vi "testSourceTree2.vi"() -> ()   [LabVIEW 2018]
panel:
  out "数値: 0から1":dbl
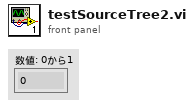
[diagram p1: front panel]
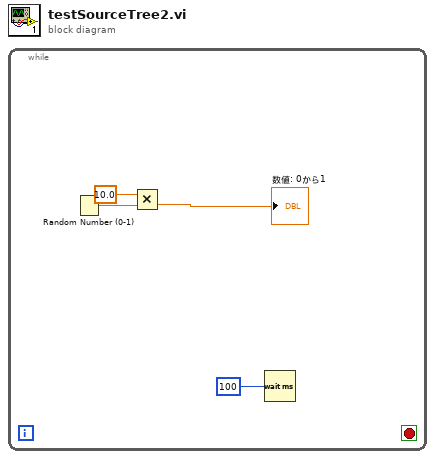
[diagram p0: block diagram]
diagram:
  n1 = while {
    stop <- _ stop-if-true
    n2 = Random Number (0-1)() -> (number: 0 to 1=w4:dbl)
    n3 = Multiply(x=10.0, y=w4) -> (x*y=→"数値: 0から1":dbl)
    n4 = Wait (ms)(milliseconds to wait=100) -> ()  [unwired: 1 out]
  }
